vi "SE Channel Number Adjustment.vi"(10 "Channels In":i32[](array[numeric])) -> (2 "Channels Out":i32[](array[numeric]))   [LabVIEW 2020]
panel:
  # "This VI simply changes any 199s to 31s.  With future driver and firmware versions, 199 will\nbe valid for all devices, but this VI changes 199s to 31s just in case."
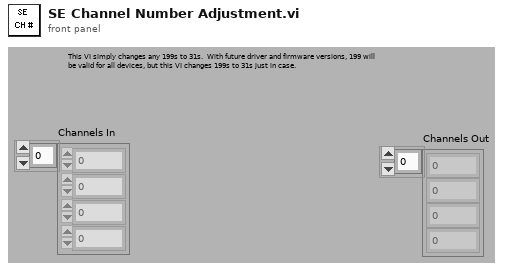
[diagram p1: front panel]
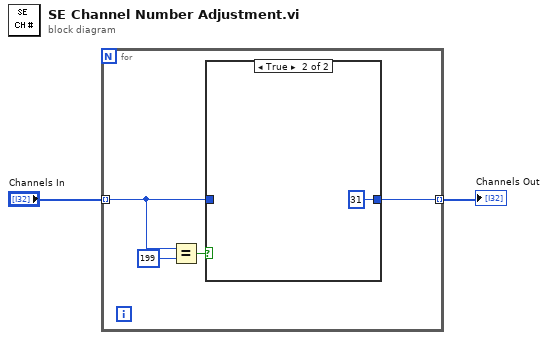
[diagram p0: block diagram]
diagram:
  n1 = for {
    tunnel: "Channels In" -> [w4] mode=indexing
    tunnel: [w3] -> w1 mode=indexing
    n2 = Equal?(x=w4, y=199) -> (x = y?=w6:bool)
    n3 = case shown="True" w6 {
      tunnel: w4 -> [w7 _]
      tunnel: [w7 31 ("Channel #")] -> w3
      frame False {
      }
      frame True {
      }
    }
  }
  "Channels Out" <- w1
